vi "Type.vi"(11 "Indicator in":refnum<class "Indicator.lvclass">) -> (2 "Type":string, 3 "Indicator out":refnum<class "Indicator.lvclass">)   [LabVIEW 2020, in "VolatusGUI.lvlib" / "Indicator.lvclass"]
uses:
  Indicator.lvclass
  Indicator.lvclass/Indicator.ctl
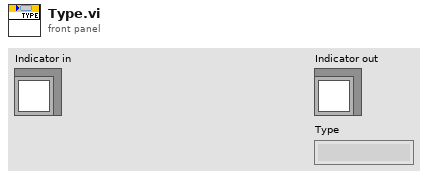
[diagram p1: front panel]
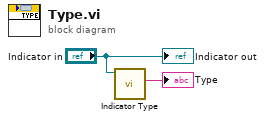
[diagram p0: block diagram]
diagram:
  n1 = call-dynamic "Indicator Type.vi"("Indicator in"="Indicator in") -> ("Indicator Type"=→"Type":string)  [unwired: 10 in]
  "Indicator out" <- "Indicator in"
